vi "OneEpoch.vi"() -> ()   [LabVIEW 2018]
uses:
  GlobalVariables/GlobalStop.vi
panel:
  in  "Control Panel":T1(tab)
  in  "Filename":path=path "test.lvm"
  in  "Tolerance Range (in decimal, not %)":dbl=0.15 format="%#_13g"
  in  "Power Supply VISA resource name":refnum<visa-resource-name>
  in  "Serial Port for Arduino":refnum<visa-resource-name>="N/A"
  in  "Designated Garbage Pin":i32
  in  "ADC Sampling Rate":dbl=10000.0 format="%0.2f"
  in  "Delay Time (s)":dbl=0.4
  in  "Set Max Current for FP":dbl=0.25 format="%#_13g"
  out "Actual Binary\nOutput":bool[](array[boolean])
  out "Target binary output":bool[](array[boolean])
  out "Current output":dbl
  out "Current (mA) level\nfor output pins":dbl[](array[numeric])
  out "Beginning Time Stamp":timestamp
  out "Pin Combination":i32
  out "RMSR":dbl
  out "Power Supply Error":string=" INSTRUCTIONS:\r\rNormal Use:  When using subVIs that incorporate the error in/error out (or error I/O) structure, place this handler where you want to inform the user of an error, typically at the end of the I/O data path, as the last action of the program.  If the error in error? is ERROR, the handler creates a message describing the error and its source.  If the type of dialog = 1 (default), the message is displayed to the user, who can only acknowedge it.  If the type = 2, the user can acknowledge the message or abort execution; aborting a program with active I/O is not recommended.  If the type = 0, no message is displayed; this is used to process the error programmatically, and the error out cluster elements are wired to individual terminals for that reason.  \r\rOther Use:\n\r\nlocal testing.  To test the error code of a subVI or function that does not have the error I/O structure, you can wire its error code and a source string to the local error code and error source inputs.  If error in error? indicates no error and error code is not equal to 0, the local code and source are substituted for the error in values, and error? is set TRUE (ERROR)."
  out "DAQ Error":string=" INSTRUCTIONS:\r\rNormal Use:  When using subVIs that incorporate the error in/error out (or error I/O) structure, place this handler where you want to inform the user of an error, typically at the end of the I/O data path, as the last action of the program.  If the error in error? is ERROR, the handler creates a message describing the error and its source.  If the type of dialog = 1 (default), the message is displayed to the user, who can only acknowedge it.  If the type = 2, the user can acknowledge the message or abort execution; aborting a program with active I/O is not recommended.  If the type = 0, no message is displayed; this is used to process the error programmatically, and the error out cluster elements are wired to individual terminals for that reason.  \r\rOther Use:\n\r\nlocal testing.  To test the error code of a subVI or function that does not have the error I/O structure, you can wire its error code and a source string to the local error code and error source inputs.  If error in error? indicates no error and error code is not equal to 0, the local code and source are substituted for the error in values, and error? is set TRUE (ERROR)."
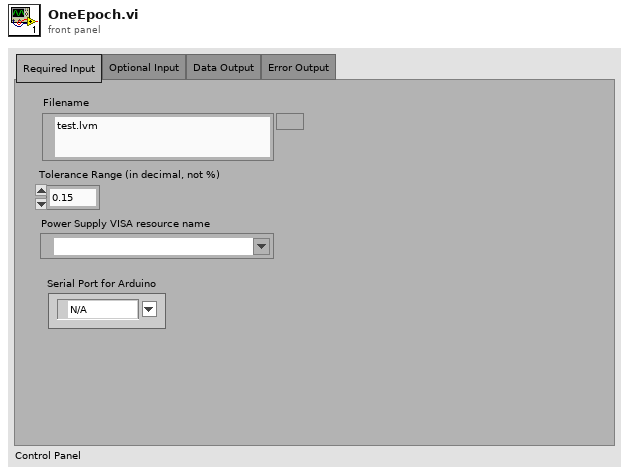
[diagram p1: front panel]
types:
  T1 = enum32{"Required Input", "Optional Input", "Data Output", "Error Output"}
  T2 = typedef "LMH-LINX.lvlib/LINX Ref.ctl" = cluster{"IO":T3, "Interface":T4, "LINX Device Config":T5}
  T3 = typedef "LMH-LINX.lvlib/Platform.ctl" = enum16{"Remote", "Local"}
  T4 = typedef "LMH-LINX.lvlib/Interface.ctl" = enum16{"Serial", "TCP"}
  T5 = typedef "LMH-LINX.lvlib/Device.lvlib/LINX Device Config.ctl" = cluster{"Interface":T4, "COM Port":refnum<visa-resource-name>, "TCP Configuration":T6, "Device Family":u8, "Device ID":u8, "Device Name":string, "TCP Ref":refnum<k5>, "Channels":T7}
  T6 = typedef "LMH-LINX.lvlib/Device.lvlib/TCP Config.ctl" = cluster{"IP Address":string, "Port":u16}
  T7 = typedef "LMH-LINX.lvlib/Channels.ctl" = cluster{"DI":u8[], "DO":u8[], "AI":u8[], "AO":u8[], "PWM":u8[], "QE":u8[], "UART":u8[], "I2C 2":u8[], "SPI":u8[], "CAN":u8[], "Servo":u8[], "AI Ref (V)":dbl, "AI Resolution (Bits)":u8, "AO Ref (V)":dbl, "AO Resolution (Bits)":u8}
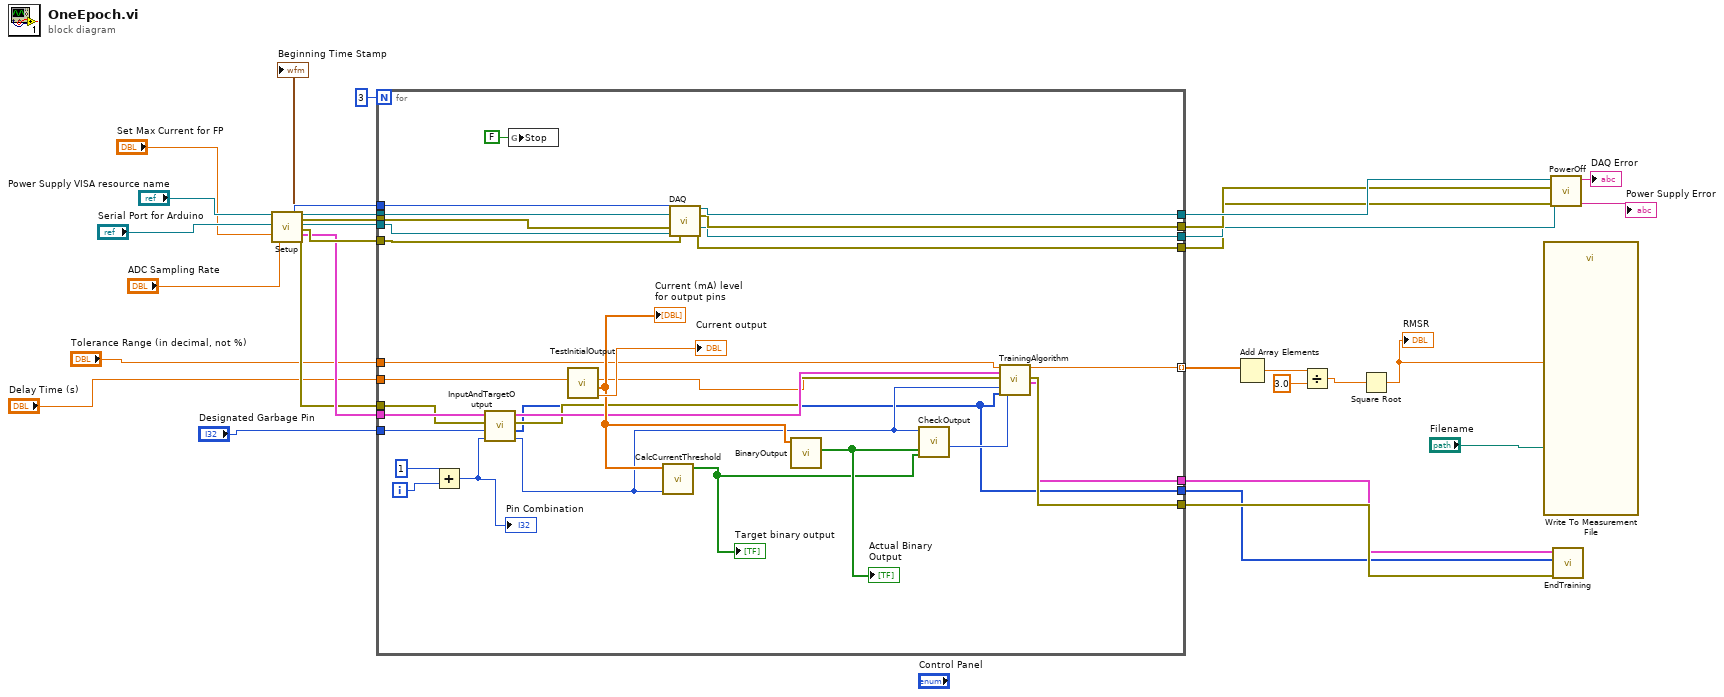
[diagram p0: block diagram]
diagram:
  n1 = call "Setup.vi"("Power Supply VISA resource name"="Power Supply VISA resource name", "Serial Port for Arduino"="Serial Port for Arduino", "Set Max Current for FP"="Set Max Current for FP", "ADC Sampling Rate"="ADC Sampling Rate") -> ("Sample Length for ADC mean 2"=w25:i32, "Beginning Time Stamp"=→"Beginning Time Stamp":timestamp, "DAQ Task Out"=w29:refnum<k21>, "DAQ Error Out"=w28:errorcluster, "VISA resource name out"=w27:refnum<visa-resource-name>, "Power Supply Error Out"=w26:errorcluster, "LINX Resource"=w24:T2, "Arduino Error Out"=w23:errorcluster)  [unwired: 8 in]
  n2 = for {
    N: 3 -> [_]
    tunnel: "Designated Garbage Pin" -> [w59]
    tunnel: w29 -> [w54]
    tunnel: w28 -> [w55]
    tunnel: w27 -> [w56]
    tunnel: w26 -> [w57]
    tunnel: w25 -> [w53]
    tunnel: w24 -> [w52]
    tunnel: w23 -> [w51]
    tunnel: "Tolerance Range (in decimal, not %)" -> [w42]
    tunnel: [w41] -> w16
    tunnel: [w40] -> w15
    tunnel: [w39] -> w14
    tunnel: [w38] -> w13
    tunnel: [w37] -> w10
    tunnel: [w36] -> w9
    tunnel: [w35] -> w8 mode=indexing
    tunnel: [w34] -> w2
    tunnel: "Delay Time (s)" -> [w33]
    i -> [w62]
    n3 = Add(x=1, y=w62) -> (x+y=w60:i32)
    "Pin Combination" <- w60
    n4 = call "InputAndTargetOutput.vi"("Decimal Input into\nLogic Block"=w60, "Designated Garbage Pin"=w59, "Error In"=w51, "LINX Resource Input"=w52) -> ("Target Output"=w46:u32, "Arduino Digital Outputs 2"=w34:u8[], "Error Out"=w44:errorcluster, "LINX Resource Output"=w45:T2)  [unwired: 2 in, 2 out]
    n5 = global write "GlobalStop.vi" "Stop"(FALSE ("Stop")) -> ()
    n6 = call "TestInitialOutput.vi"("Delay Time (s)"=w33) -> ("Current output (mA)"=→"Current output":dbl, "Current (mA) level\nfor output pins"=w50:dbl[], "Delay Time"=w43:dbl)  [unwired: 8 in]
    "Current (mA) level\nfor output pins" <- w50
    n7 = call "CalcCurrentThreshold.vi"("Target Decimal Output"=w46, "Current of Output Pins"=w50) -> ("Target binary output"=w48:bool[])  [unwired: 8 in, 1 out]
    "Target binary output" <- w48
    n8 = call "DAQ.vi"("sample length"=w53, "task/channels in"=w54, "error in"=w55, "VISA resource name out"=w56, "error out"=w57) -> ("task out"=w41:refnum<k21>, "error out 2"=w40:errorcluster, "VISA resource name out 2"=w39:refnum<visa-resource-name>, "error out 3"=w38:errorcluster)  [unwired: 7 in]
    n9 = call "BinaryOutput.vi"("Current Level of Output Pins 2"=w50) -> ("Actual Binary\nOutput"=w49:bool[])  [unwired: 9 in, 1 out]
    "Actual Binary\nOutput" <- w49
    n10 = call "CheckOutput.vi"("Target Binary Output"=w48, "Actual Binary Output"=w49, "Expected Output Pin"=w46) -> ("Pin to Train"=w47:i32)  [unwired: 7 in, 1 out]
    n11 = call "TrainingAlgorithm.vi"("Tolerance Range (in decimal, not %)"=w42, "LINX Resource"=w45, "Error In"=w44, "Delay Time (s)"=w43, "Target \nOutput"=w46, "Arduino Digital Outputs"=w34, "Most Erroneous\nPin Index Number"=w47) -> ("[unwanted/total]^2"=w35:dbl, "Error Out"=w37:errorcluster, "LINX Resource 2"=w36:T2)  [unwired: 10 in]
  }
  n12 = Add Array Elements(numeric array=w8) -> (sum=w7:dbl)
  n13 = Divide(x=w7, y=3.0) -> (x/y=w5:dbl)
  n14 = Square Root(x=w5) -> (sqrt(x)=w4:dbl)
  "RMSR" <- w4
  n15 = call "Write To Measurement File"("Signals"=w4, "Filename"="Filename") -> ()  [unwired: 15 in, 3 out]
  n16 = call "PowerOff.vi"("Power Supply Error IN"=w13, "VISA resource name"=w14, "DAQ Error In"=w15, "DAQ Channels"=w16) -> ("Power Supply Error"=→"Power Supply Error":string, "DAQ Error"=→"DAQ Error":string)  [unwired: 6 in]
  n17 = call "EndTraining.vi"("Error In"=w10, "DO Channels"=w2, "LINX Resource"=w9) -> ()  [unwired: 9 in]
